vi "getMatrixStatus.vi"() -> (1 "Meas Matrices Filled?":bool[](array[boolean]))   [LabVIEW 2012]
uses:
  bin/OVA32.dll
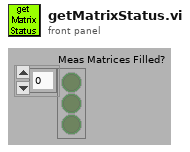
[diagram p1: front panel]
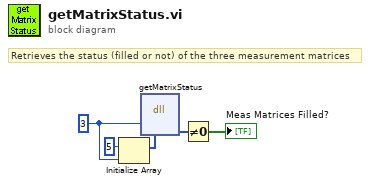
[diagram p0: block diagram]
diagram:
  w3 = u32 3 ("numMatrices")
  # "Retrieves the status (filled or not) of the three measurement matrices"
  n1 = Initialize Array(u8 5 ("Element Data"), w3) -> (w2:u8[])
  n2 = dll-call lib="C:/_src/OVA5000_DSP_falcon/Software/LabVIEW/OVA/SDK/OVA_5000_SDK_v5.14.3/bin/OVA32.dll" fn="getMatrixStatus"("numMatrices"=w3, "filled"=w2) -> ("filled"=w5:u8[])  [unwired: 5 in, 2 out]
  n3 = Not Equal To 0?(x=w5) -> (x != 0?=→"Meas Matrices Filled?":bool[])
